vi "Euler Angles To Direction Cosines.vi"(11 "Euler Angles":cluster{"phi":dbl, "theta":dbl, "psi":dbl}) -> (0 "error":i32, 3 "Direction Cosines":dbl[][](array[numeric]))   [LabVIEW 2010, in "NI_AALPro.lvlib"]
doc: "Converts Euler angles into a 3-by-3 matrix of direction cosines."
uses:
  NI_AALPro.lvlib
  lvanlys.dll
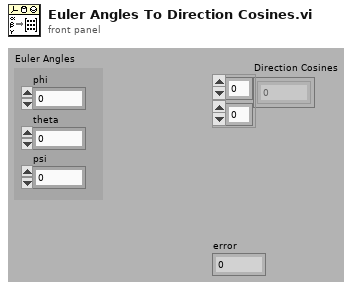
[diagram p1: front panel]
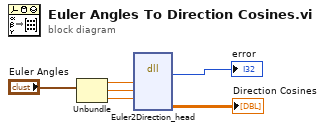
[diagram p0: block diagram]
diagram:
  n1 = Unbundle("Euler Angles") -> ("phi"=w5:dbl, "theta"=w4:dbl, "psi"=w3:dbl)
  n2 = dll-call lib="C:/Program Files/National Instruments/LabVIEW 2010/resource/lvanlys.*" fn="Euler2Direction_head"("phi"=w5, "theta"=w4, "psi"=w3) -> (→"error":i32, "direction"=→"Direction Cosines":dbl[][])  [unwired: 7 in, 2 out]
